vi "DAQmx_Pulse_CountContinuous.vi"(10 "CI.CountEdges.Term":tag="/Dev1/PFI0", 11 "counter":tag="Dev1/ctr0") -> ()   [LabVIEW 2025]
uses:
  <vilib>/DAQmx/read.llb/DAQmx Read (Counter U32 1Chan 1Samp).vi
  <vilib>/DAQmx/create/channels.llb/DAQmx Create Channel (CI-Count Edges).vi
  <vilib>/DAQmx/configure/timing.llb/DAQmx Timing (Sample Clock).vi
  <vilib>/DAQmx/miscellaneous.llb/DAQmx Fill In Error Info.vi
  <resource>/objmgr/daqmx.rc
panel:
  in  "stop":bool
  out "Number of Counted Pulses":u32
  in  "CI.CountEdges.ActiveEdge":i32(ring)=10280 items=["Rising"=10280, "Falling"=10171]
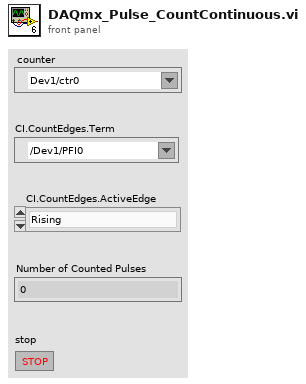
[diagram p1: front panel]
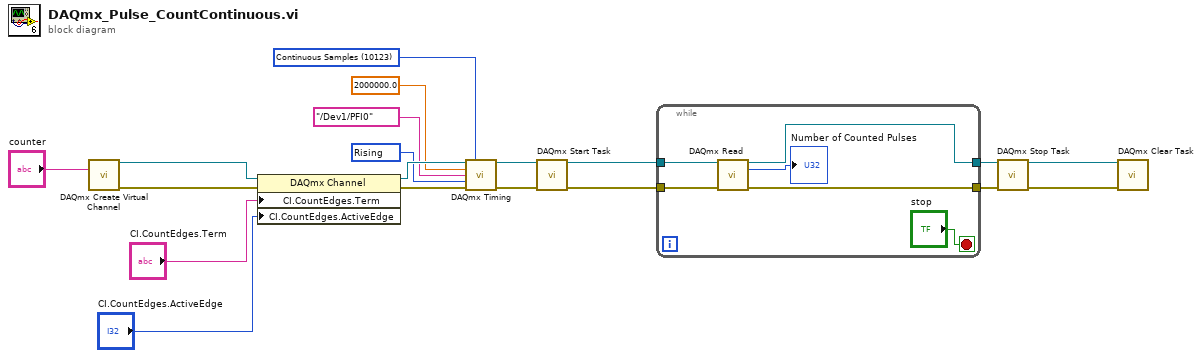
[diagram p0: block diagram]
diagram:
  w2 = 10280 items=["Rising"=10280, "Falling"=10171] ("active edge")
  w4 = 10123 items=["Finite Samples"=10178, "Continuous Samples"=10123, "Hardware Timed Single Point"=12522] ("sample mode")
  n1 = call-poly <vilib>:"DAQmx Create Virtual Channel.vi"("counter"="counter") -> ("task out"=w18:refnum<k21>, "error out"=w17:errorcluster)  [unwired: 13 in]
  n2 = property class="DAQmx Channel"(reference=w18, error in=w17, "CI.CountEdges.Term"="CI.CountEdges.Term", "CI.CountEdges.ActiveEdge"="CI.CountEdges.ActiveEdge") -> (reference out=w6:refnum<k21>, error out=w8:errorcluster)
  n3 = call-poly <vilib>:"DAQmx Timing.vi"("task/channels in"=w6, "sample mode"=w4, "rate"=2000000.0, "source"=tag "/Dev1/PFI0", "active edge"=w2, "error in"=w8) -> ("task out"=w5:refnum<k21>, "error out"=w7:errorcluster)  [unwired: 8 in]
  n4 = call <vilib>:"DAQmx Start Task.vi"("task/channels in"=w5, "error in"=w7) -> ("task out"=w15:refnum<k21>, "error out"=w14:errorcluster)  [unwired: 12 in]
  n5 = while {
    tunnel: w15 -> [w25]
    tunnel: w14 -> [w24]
    tunnel: [w23] -> w13
    tunnel: [w22] -> w12
    stop <- "stop" stop-if-true
    n6 = call-poly <vilib>:"DAQmx Read.vi"("task/channels in"=w25, "error in"=w24) -> ("task out"=w23:refnum<k21>, "data"=→"Number of Counted Pulses":u32, "error out"=w22:errorcluster)  [unwired: 11 in]
  }
  n7 = call <vilib>:"DAQmx Stop Task.vi"("task/channels in"=w13, "error in"=w12) -> ("task out"=w11:refnum<k21>, "error out"=w10:errorcluster)  [unwired: 12 in]
  n8 = call <vilib>:"DAQmx Clear Task.vi"("task in"=w11, "error in"=w10) -> ()  [unwired: 13 in, 1 out]
